vi "FM Demod Sound Card.vi"() -> ()   [LabVIEW 2015]
uses:
  <vilib>/sound2/lvsound2.llb/Sound Data Format.ctl
  <vilib>/sound2/lvsound2.llb/Sampling Mode.ctl
  <vilib>/sound2/lvsound2.llb/Sound Output Write (DBL Single).vi
  <vilib>/measure/maspectr.llb/FFT Power Spectrum and PSD for 1 Chan.vi
  <instrlib>/niUSRP/niUSRP Fetch Rx Data (CDB Cluster).vi
  <vilib>/measure/maresamp.llb/Resample Waveform (single shot).vi
  <vilib>/addons/Modulation/niAMT.lvlib
  <vilib>/measure/NI_MAPro.lvlib
panel:
  in  "Averaging Mode":T1(ring)
  in  "Sound On":bool
  in  "Cursor.Visible":bool
  out "FM Demodulated":waveform(dbl)(graph)={"t0"=timestamp(8822.67583072 s since 1904-01-01), "dt"=2.2675736961451248e-05, "Y"=[]}
  out "Frequency Spectrum":cluster{"f0":dbl, "df":dbl, "magnitude":dbl[]}(graph)={"f0"=0.0, "df"=5.0, "magnitude"=[]}
  in  "Receiving Parameters":T2={"Rx IQ Sampling\nRate [s/sec]"=200000.0, "Rx\nFrequency [Hz]"=94700000.0, "Rx Gain [dB]"=20.0, "Rx Antenna"="RX1"} {"Rx Gain [dB]" format="%#.6p"; "Rx\nFrequency [Hz]" format="%#.6p"; "Rx IQ Sampling\nRate [s/sec]" format="%#.6p"}
  in  "stop":bool
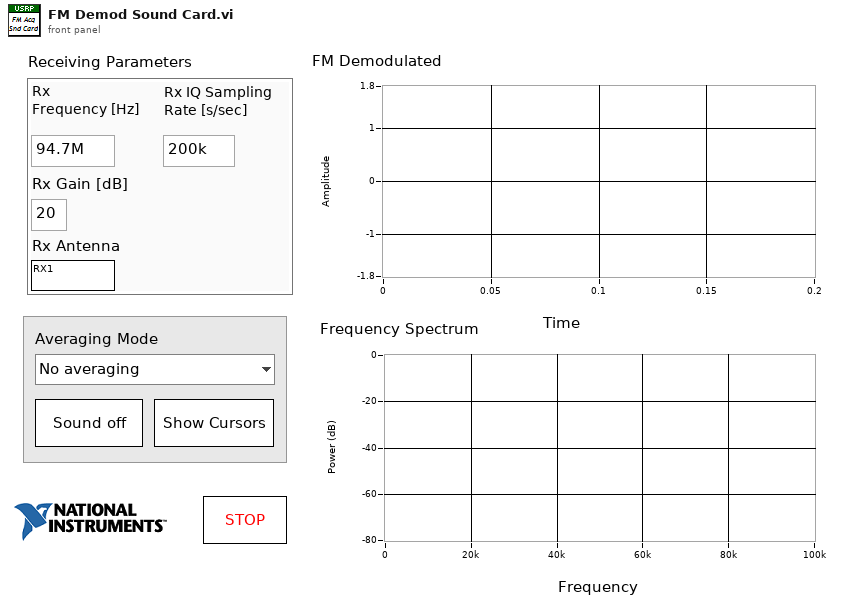
[diagram p1: front panel]
types:
  T1 = enum16{"No averaging", "Vector averaging", "RMS averaging", "Peak hold"}
  T2 = cluster{"Rx IQ Sampling\nRate [s/sec]":dbl, "Rx\nFrequency [Hz]":dbl, "Rx Gain [dB]":dbl, "Rx Antenna":string}
  T3 = typedef "Sampling Mode.ctl" = i32
  T4 = typedef "Sound Data Format.ctl" = cluster{"sample rate (S/s)":dbl, "number of channels":i32, "bits per sample":i32}
  T5 = typedef "Sound Output Task ID.ctl" = u32
  T6 = cluster{"averaging mode":enum16{"No averaging", "Vector averaging", "RMS averaging", "Peak hold"}, "weighting mode":enum16{"Linear", "Exponential"}, "number of averages":u32}
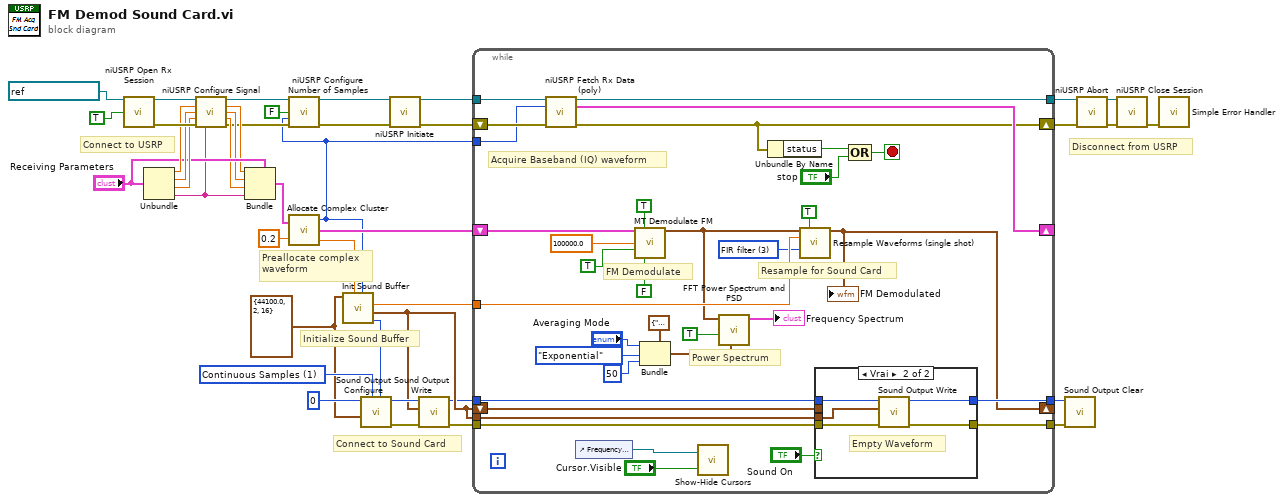
[diagram p0: block diagram]
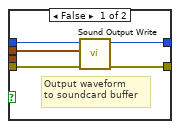
[diagram p2: hidden frame]
diagram:
  w29 = T3 1 items=["Finite Samples", "Continuous Samples"] ("sample mode")
  w22 = T4 {"sample rate (S/s)"=44100.0, "number of channels"=2, "bits per sample"=16} ("sound format")
  # "Disconnect from USRP"
  # "Initialize Sound Buffer"
  # "Preallocate complex \nwaveform"
  # "Connect to USRP"
  # "Connect to Sound Card"
  n1 = call <instrlib>:"niUSRP Open Rx Session.vi"("device names"=refnum<k15> "192.168.10.2", "reset"=TRUE) -> ("session handle out"=w17:refnum<k15>, "error out"=w16:errorcluster)  [unwired: 12 in]
  n2 = Unbundle("Receiving Parameters") -> ("Rx IQ Sampling\nRate [s/sec]"=w15:dbl, "Rx\nFrequency [Hz]"=w14:dbl, "Rx Gain [dB]"=w13:dbl, "Rx Antenna"=w11:string)
  n3 = call <instrlib>:"niUSRP Configure Signal.vi"("session handle"=w17, "IQ rate"=w15, "carrier frequency"=w14, "gain"=w13, "error in (no error)"=w16, "active antenna"=w11) -> ("session handle out"=w6:refnum<k15>, "coerced IQ rate"=w8:dbl, "coerced carrier frequency"=w9:dbl, "coerced gain"=w10:dbl, "error out"=w5:errorcluster)  [unwired: 5 in]
  n4 = Bundle(cluster="Receiving Parameters", "Rx IQ Sampling\nRate [s/sec]"=w8, "Rx\nFrequency [Hz]"=w9, "Rx Gain [dB]"=w10, "Rx Antenna"=w11) -> (w7:T2)
  n5 = call "Allocate Complex Cluster.vi"("Seconds\nper Frame"=0.2 ("Seconds\nper Frame"), "Actual Rx Parameters"=w7) -> ("Rx IQ Sampling\nRate [s/sec]"=w23:dbl, "Allocated Cluster"=w36:cluster{"t0":dbl, "dt":dbl, "Y":cdb[]}, "Number of Samples"=w2:i32)
  n6 = call <instrlib>:"niUSRP Configure Number of Samples.vi"("session handle"=w6, "number of samples is finite"=FALSE, "number of samples"=w2, "error in (no error)"=w5) -> ("session handle out"=w4:refnum<k15>, "error out"=w1:errorcluster)  [unwired: 10 in]
  n7 = call "Init Sound Buffer.vi"("Number of Samples"=w2, "Rx IQ Sampling\nRate [s/sec]"=w23, "sound format"=w22) -> ("Samples/ch"=w24:i32, "Allocated Waveform"=w26:waveform(dbl), "dt"=w27:dbl)  [unwired: 6 in]
  n8 = call <vilib>:"Sound Output Configure.vi"("number of samples/ch"=w24, "sample mode"=w29, "sound format"=w22, "device ID"=u32 0 ("Sound Card ID")) -> ("error out"=w20:errorcluster, "task ID"=w30:T5)  [unwired: 6 in]
  n9 = call <instrlib>:"niUSRP Initiate.vi"("session handle"=w4, "error in (no error)"=w1) -> ("session handle out"=w41:refnum<k15>, "error out"=w31:errorcluster)  [unwired: 12 in]
  n10 = call-poly <vilib>:"Sound Output Write.vi"("error in (no error)"=w20, "data"=w26, "task ID"=w30) -> ("error out"=w19:errorcluster, "task ID out"=w25:T5)  [unwired: 7 in]
  n11 = while {
    tunnel: [w67] -> w40
    shift-right: [w57] -> w39
    shift-left: w31 -> [w66]
    tunnel: [w72] -> w33
    tunnel: w27 -> [w55]
    tunnel: w41 -> [w68]
    shift-right: [w56] -> _
    shift-left: w26 -> [w69]
    shift-right: [w60] -> _
    shift-left: w36 -> [w65]
    tunnel: w26 -> [w62]
    tunnel: w25 -> [w58]
    tunnel: w19 -> [w44]
    tunnel: [w43] -> w18
    tunnel: w2 -> [w42]
    stop <- w73 stop-if-true
    w45 = u16 3 items=["coerce", "linear", "spline", "FIR filter"] ("interpolation mode")
    # "Resample for Sound Card"
    # "Power Spectrum"
    # "Acquire Baseband (IQ) waveform"
    # "FM Demodulate"
    n12 = call-poly <instrlib>:"niUSRP Fetch Rx Data (poly).vi"("session handle"=w68, "number of samples"=w42, "error in (no error)"=w66) -> ("session handle out"=w67:refnum<k15>, "data"=w60:cluster{"t0":dbl, "dt":dbl, "Y":cdb[]}, "error out"=w57:errorcluster)  [unwired: 9 in, 1 out]
    n13 = control-ref of="Frequency Spectrum"() -> (w63:refnum<vi>)
    n14 = call <vilib>:"MT Demodulate FM.vi"("FM modulated waveform"=w65, "reset? (F)"=TRUE, "FM deviation (Hz)"=100000.0, "carrier correction? (F)"=TRUE, "remove transient when reset? (F)"=FALSE) -> ("FM demodulated waveform"=w47:waveform(dbl))  [unwired: 8 in, 2 out]
    n15 = Bundle(cluster=T6 {"averaging mode"=enum."No averaging", "weighting mode"=enum."Exponential", "number of averages"=10} ("averaging parameters"), "averaging mode"="Averaging Mode", "weighting mode"=enum16{"Linear", "Exponential"}."Exponential", "number of averages"=u32 50) -> (w49:T6)
    n16 = call "Show-Hide Cursors.vi"("Cursors On?(F)"="Cursor.Visible", "WFGraph Refnum"=w63) -> ()  [unwired: 2 in]
    n17 = call-poly <vilib>:"FFT Power Spectrum and PSD.vi"("averaging parameters"=w49, "dB On (F)"=TRUE, "time signal"=w47) -> ("Power Spectrum / PSD"=→"Frequency Spectrum":cluster{"f0":dbl, "df":dbl, "magnitude":dbl[]})  [unwired: 5 in, 3 out]
    n18 = Unbundle By Name(w57) -> ("status"=w59:bool)
    n19 = call-poly <vilib>:"Resample Waveforms (single shot).vi"("waveform in"=w47, "open interval? (F)"=TRUE, "dt"=w55, "interpolation mode"=w45) -> ("resampled waveform out"=w56:waveform(dbl))  [unwired: 8 in, 3 out]
    "FM Demodulated" <- w56
    n20 = case shown="Vrai" "Sound On" {
      tunnel: [w81 w86] -> w72
      tunnel: w69 -> [w80 _]
      tunnel: w62 -> [_ w85]
      tunnel: w58 -> [w79 w84]
      tunnel: w44 -> [w78 w83]
      tunnel: [w77 w82] -> w43
      frame False {
        # "Output waveform \nto soundcard buffer"
        n21 = call-poly <vilib>:"Sound Output Write.vi"("error in (no error)"=w78, "data"=w80, "task ID"=w79) -> ("error out"=w77:errorcluster, "task ID out"=w81:T5)  [unwired: 7 in]
      }
      frame True {
        # "Empty Waveform"
        n22 = call-poly <vilib>:"Sound Output Write.vi"("error in (no error)"=w83, "data"=w85, "task ID"=w84) -> ("error out"=w82:errorcluster, "task ID out"=w86:T5)  [unwired: 7 in]
      }
    }
    n23 = Compound Arithmetic op=OR(w59, "stop") -> (w73:bool)
  }
  n24 = call <vilib>:"Sound Output Clear.vi"("error in (no error)"=w18, "task ID"=w33) -> ()  [unwired: 9 in, 1 out]
  n25 = call <instrlib>:"niUSRP Abort.vi"("session handle"=w40, "error in (no error)"=w39) -> ("session handle out"=w38:refnum<k15>, "error out"=w37:errorcluster)  [unwired: 12 in]
  n26 = call <instrlib>:"niUSRP Close Session.vi"("session handle"=w38, "error in (no error)"=w37) -> ("error out"=w21:errorcluster)  [unwired: 13 in]
  n27 = call <vilib>:"Simple Error Handler.vi"("error in (no error)"=w21) -> ()  [unwired: 4 in, 5 out]
